vi "Configure Power Analysis (Quality).vi"(8 "error in (no error)":errorcluster, 10 "Measurement Type (0: Power Factor)":i32(ring) items=["Power Factor", "Real Power", "Apparent Power", "Reactive Power", "Crest Factor", "Phase Angle"], 11 "VISA resource name":refnum<visa-resource-name>) -> (0 "error out":errorcluster, 3 "VISA resource name out":refnum<visa-resource-name>)   [LabVIEW 2015, in "Agilent 2000 3000 X-Series.lvlib"]
doc: "Applies a specific power quality analysis type.\n\n<B>Note(s):</B>\nUse <B>Read Measurement (Quality Power Analysis).vi</B> to read the result of this power analysis."
uses:
  <instrlib>/Agilent 2000 3000 X-Series/Agilent 2000 3000 X-Series.lvlib
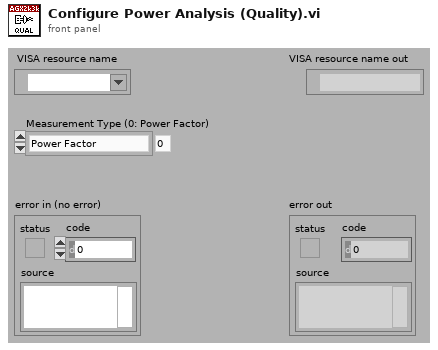
[diagram p1: front panel]
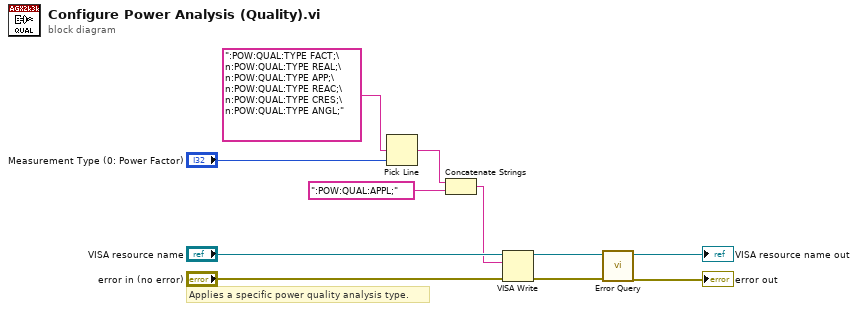
[diagram p0: block diagram]
diagram:
  # "Applies a specific power quality analysis type."
  n1 = Pick Line(multi-line string=":POW:QUAL:TYPE FACT;\n:POW:QUAL:TYPE REAL;\n:POW:QUAL:TYPE APP;\n:POW:QUAL:TYPE REAC;\n:POW:QUAL:TYPE CRES;\n:POW:QUAL:TYPE ANGL;", line index="Measurement Type (0: Power Factor)") -> (output string=w3:string)  [unwired: 1 out]
  n2 = Concatenate Strings(w3, ":POW:QUAL:APPL;") -> (w1:string)
  n3 = VISA Write(VISA resource name="VISA resource name", write buffer=w1, error in (no error)="error in (no error)") -> (VISA resource name out=w7:refnum<visa-resource-name>, error out=w6:errorcluster)  [unwired: 1 out]
  n4 = call <instrlib>:"Error Query.vi"("error in (no error)"=w6, "VISA resource name"=w7) -> ("error out"=→"error out":errorcluster, "VISA resource name out"=→"VISA resource name out":refnum<visa-resource-name>)  [unwired: 8 out]
